vi "NewLPF2CodeTest.vi"() -> ()   [LabVIEW 2016]
uses:
  VIs/uPythonX/uPythonX.xctl
panel:
  in  "LPF2Class.py":T1(xcontrol)={"VISA Refnum in"="ASRL12::INSTR", "Python Code"="import machine, utime, gc\nimport math, struct\nimport utime,pyb\n\nCMD_Type = 0x40   # set sensor type command\nCMD_Mode = 0x49   # set mode type command\nCMD_Baud = 0x52   # set the transmission baud rate\nCMD_Vers = 0x5F   # set the version number\nCMD_ModeInfo = 0x80  # name command\n\nNAME,RAW,Pct,SI,SYM,FCT, FMT = 0x0,0x1,0x2,0x3,0x4,0x5, 0x80\nDATA8,DATA16,DATA32,DATAF = 0,1,2,3  # Data type codes\nABSOLUTE,RELATIVE,DISCRETE = 16,8,4\n\n# Name, Format [# datasets, type, figures, decimals], raw [min,max], Percent, SI, Symbol,functionMap, view\nmode0 = ['LPF2-DETECT',[1,DATA8,3,0],[0,10],[0,100],[0,10],'',[ABSOLUTE,0],True]\nmode1 = ['LPF2-COUNT',[1,DATA32,4,0],[0,100],[0,100],[0,100],'CNT',[ABSOLUTE,0],True]\nmode2 = ['LPF2-CAL',[3,DATA16,3,0],[0,1023],[0,100],[0,1023],'RAW',[ABSOLUTE,0],False]\nmodes = [mode0,mode1,mode2]\n\nclass LPF2(object):\n     def __init__(self, uartChannel, txPin, rxPin, timer = 4, freq = 5):\n          self.txPin = txPin\n          self.rxPin = rxPin\n          self.uart = machine.UART(uartChannel)\n          self.txTimer = timer\n          self.connected = False\n          self.payload = bytearray([])\n          self.freq = freq\n          self.oldbuffer =  bytes([])\n\n     def load_payload(self,data):\n          value = (data & 0xFF)\n          self.payload = bytes([0xC0, value, 0xFF ^ 0xC0 ^ value])\n          \n     def sendCall(self, timerInfo):\n          if self.connected:\n               size = self.writeIt(self.payload)\n               if not size: self.connected = False\n\n     def writeIt(self,array):\n          #print(binascii.hexlify(array))\n          return self.uart.write(array)\n          \n     def readIt2(self):\n          reply = b''\n          if self.uart.any() > 0:\n               reply = self.uart.read(self.uart.any())\n          return reply\n          \n     def readIt(self):\n          if self.uart.any() == 0:    # if nothing is there then leave\n               return b''\n          if not self.waitFor(b'\\x02'):\n               return b''\n          status, data = self.waitFor(b'\\x02')\n          if not status:    # make sure it is long enough to give data\n               return b''\n          #data = data[0:-1] if (data[-1] == 2) else data\n          loc = data.find(b'F')\n          if (loc >= 0) and (len(data) > 5):       \n               mode = data[1]\n               something = data[2]\n               chksm = data[-1]\n               counter = data[3]\n               payload = data[4:-1]\n               chksm2 = 0xFF ^ counter\n               for i in payload:\n                    chksm2 ^= i\n               if not(chksm == chksm2):\n                    print('checksum error   read %d, measured %d' % (chksm,chksm2))\n          else:\n               payload = b''\n          return data #payload\n\n     def waitFor (self, char, timeout = 2):\n          starttime = utime.time()\n          currenttime = starttime\n          status = False\n          buffer = self.oldbuffer\n          while (currenttime-starttime) < timeout:\n               utime.sleep_ms(5)\n               data = self.uart.read(self.uart.any())   #self.readIt()\n               buffer += data\n               if data.find(char) >= 0:\n                    status = True\n                    reply = buffer.split(char)\n                    buffer = reply[0]\n                    self.oldbuffer = reply[-1]   # dumps any extra readings\n                    currenttime = starttime + timeout   # stop the loop\n               else:\n                    currenttime = utime.time()\n          return status, buffer\n\n          \n     def addChksm(self,array):\n          chksm = 0\n          for b in array:\n               chksm ^= b\n          chksm ^= 0xFF\n          array.append(chksm)  \n          return array\n          \n     def init(self):\n          self.tx = machine.Pin(self.txPin, machine.Pin.OUT)\n          self.rx = machine.Pin(self.rxPin, machine.Pin.IN)\n          self.tx.value(0)\n          utime.sleep_ms(500)\n          self.tx.value(1)\n          self.uart.init(baudrate=2400, bits=8, parity=None, stop=1)\n          self.writeIt(b'\\x00')\n\n     def type(self,sensorType):\n          return self.addChksm(bytearray([CMD_Type, sensorType]))\n\n     def defineBaud(self,baud):\n          rate = baud.to_bytes(4, 'little')\n          return self.addChksm(bytearray([CMD_Baud]) + rate) \n\n     def defineVers(self,hardware,software):\n          hard = hardware.to_bytes(4, 'big')\n          soft = software.to_bytes(4, 'big')\n          return self.addChksm(bytearray([CMD_Vers]) + hard + soft)\n          \n     def padString(self,string, num, startNum):\n          reply = bytearray([startNum])  # start with name\n          reply += string\n          exp = math.ceil(math.log(len(string),2)) if len(string)>0 else 0  # find the next power of 2\n          size = 2**exp\n          exp = exp<<3\n          length = size - len(string)\n          for i in range(length):\n               reply += bytearray([0])\n          return self.addChksm(bytearray([CMD_ModeInfo | exp | num]) + reply)\n\n     def buildFunctMap(self,mode, num, Type):\n          exp = 1 << 3\n          mapType = mode[0]\n          mapOut = mode[1]\n          return self.addChksm(bytearray([CMD_ModeInfo | exp | num, Type, mapType, mapOut]))\n\n     def buildFormat(self,mode, num, Type):\n          exp = 2 << 3\n          sampleSize = mode[0] & 0xFF\n          dataType = mode[1] & 0xFF\n          figures = mode[2] & 0xFF\n          decimals = mode[3] & 0xFF\n          return self.addChksm(bytearray([CMD_ModeInfo | exp | num, Type, sampleSize, dataType,figures,decimals]))\n     \n     def buildRange(self,settings, num, rangeType):\n          exp = 3 << 3\n          minVal = struct.pack('<f', settings[0])\n          maxVal = struct.pack('<f', settings[1])\n          return self.addChksm(bytearray([CMD_ModeInfo | exp | num, rangeType]) + minVal + maxVal)\n\n     def defineModes(self,modes):\n          length = (len(modes)-1) & 0xFF\n          views = 0\n          for i in modes:\n               if (i[7]):\n                    views = views + 1\n          views = (views - 1) & 0xFF\n          return self.addChksm(bytearray([CMD_Mode, length, views]))\n          \n     def setupMode(self,mode,num):\n          self.writeIt(self.padString(mode[0],num,NAME)) # write name\n          self.writeIt(self.buildRange(mode[2], num, RAW)) # write RAW range\n          self.writeIt(self.buildRange(mode[3], num, Pct)) # write Percent range\n          self.writeIt(self.buildRange(mode[4], num, SI)) # write SI range\n          self.writeIt(self.padString(mode[5],num,SYM)) # write symbol\n          self.writeIt(self.buildFunctMap(mode[6],num, FCT)) # write Function Map\n          self.writeIt(self.buildFormat(mode[1],num, FMT)) # write format\n\n     def initialize(self):\n          self.connected = False\n          self.sendTimer = pyb.Timer(self.txTimer, freq = self.freq)  # default is 200 ms\n          self.init()\n          self.writeIt(self.type(35))  # set type to 35 \n          self.writeIt(self.defineModes(modes))  # tell how many modes \n          self.writeIt(self.defineBaud(115200))\n          self.writeIt(self.defineVers(2,2))\n\n          num = len(modes) - 1\n          for mode in reversed(modes):\n               self.setupMode(mode,num)\n               num -= 1\n               utime.sleep_ms(5)\n               \n          self.writeIt(b'\\x04')  #ACK\n          # Check for ACK reply\n          self.connected, buffer = self.waitFor(b'\\x04')\n          print('Success' if self.connected else 'Failed')\n\n          # Reset Serial to High Speed\n          # pull pin low\n          self.uart.deinit()\n          if self.connected:\n               tx = machine.Pin(self.txPin, machine.Pin.OUT)\n               tx.value(0)\n               utime.sleep_ms(10)\n               \n               #change baudrate\n               self.uart.init(baudrate=115200, bits=8, parity=None, stop=1)\n               self.load_payload(2)\n          \n               #start callback  - MAKE SURE YOU RESTART THE CHIP EVERY TIME (CMD D) to kill previous callbacks running\n               self.sendTimer.callback(self.sendCall)\n          return\n"}
  in  "Spike":T1(xcontrol)={"VISA Refnum in"="ASRL73::INSTR", "Python Code"="import hub,utime\n\nhub.port.B.info()\n\n# if info comes back with None - then you have to restart the pybaord\n\nwhile True:\n     try:\n          value = hub.port.B.device.get()[0]\n          #print(value)\n          hub.display.show(str(value))\n          #print(value)\n          if value == 9:\n               hub.port.B.device.mode(0,b'toggle')\n          utime.sleep(0.1)\n     except:\n          utime.sleep(1)\n\n'''\nhub.port.B.device.mode([(0,0),(1,0),(1,2),(3,0)])\n\nhub.port.B.device.mode(0,b'hi there')\n'''"}
  in  "Camera":T1(xcontrol)={"VISA Refnum in"="ASRL12::INSTR", "Python Code"="import gc,utime\nimport pyb, micropython\nfrom LPF2Class import LPF2\n\nmicropython.alloc_emergency_exception_buf(200)\n\nred_led=pyb.LED(1)\ngreen_led = pyb.LED(2)\nred_led.on()\n\nlpf2 = LPF2(3, 'P4', 'P5', timer = 4, freq = 5)    # OpenMV\nlpf2.initialize()\n\nvalue = 0\n\n# Loop\nwhile True:\n     if not lpf2.connected:\n          lpf2.sendTimer.callback(None)\n          red_led.on()\n          utime.sleep_ms(200)\n          lpf2.initialize()\n     else:\n          red_led.off()\n          value = value + 1 if value < 9 else 0\n          lpf2.load_payload(value)\n          data = lpf2.readIt2()\n          if len(data) > 0:\n               print(data)\n               if data.find(b'toggle')>=0:\n                    green_led.toggle()\n\n          utime.sleep_ms(200)\n\n"}
  # "Download this to your backpack"
  # "Run this on SPIKE\n(and close the window)"
  # "Edit this code"
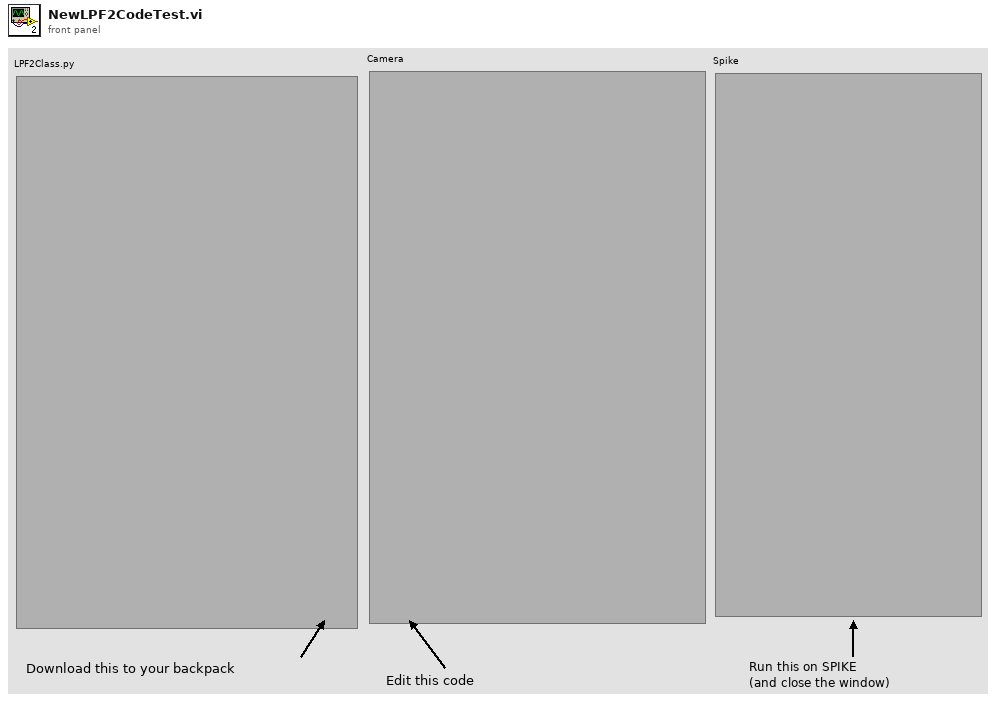
[diagram p1: front panel]
types:
  T1 = cluster{"VISA Refnum in":refnum<visa-resource-name>, "Python Code":string}
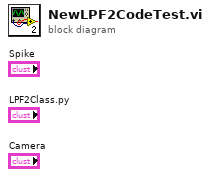
[diagram p0: block diagram]
diagram:
